vi "For contador.vi"() -> ()   [LabVIEW 2020]
panel:
  in  "stop":bool
  in  "millisecond timer value":u32
  out "Alea":dbl
  out "Numeric":i32
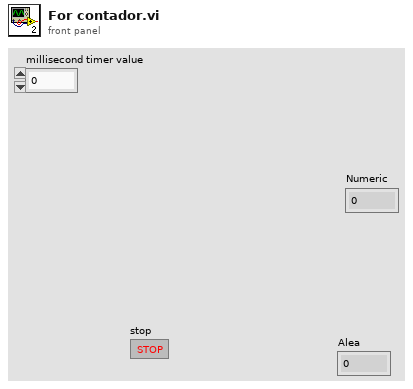
[diagram p1: front panel]
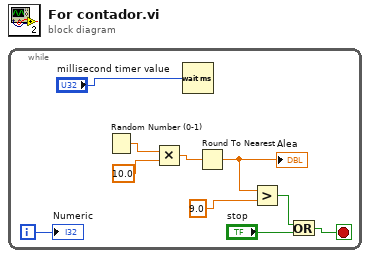
[diagram p0: block diagram]
diagram:
  n1 = while {
    i -> [w10]
    stop <- w1 stop-if-true
    n2 = Random Number (0-1)() -> (number: 0 to 1=w9:dbl)
    n3 = Multiply(x=w9, y=10.0) -> (x*y=w7:dbl)
    n4 = Wait (ms)(milliseconds to wait="millisecond timer value") -> ()  [unwired: 1 out]
    n5 = Round To Nearest(number=w7) -> (nearest integer value=w5:dbl)
    "Alea" <- w5
    n6 = Greater?(x=w5, y=9.0) -> (0:w3:bool)
    n7 = Or(x=w3, y="stop") -> (x .or. y?=w1:bool)
    "Numeric" <- w10
  }
